vi "Statistics.vi"(11 "input data":dbl[](array[numeric])=[4.507, 5.12, 4.497, 5.011, 3.613, 3.857, 5.086, 3.732, 3.995, 3.022, 4.463, 4.377]) -> ()   [LabVIEW 2018]
doc: "This example shows the results of statistical functions. There is a Histogram of all values and there is the Minimum, Maximum and Mean for each packet of data.\n\nThis example uses the following Express VIs: Simulate Signal, Create Histogram, and Statistics."
uses:
  <vilib>/Utility/file.llb/Read Delimited Spreadsheet (DBL).vi
  Instance           2 18Saved   Statistics .vi
  Instance           3 18Saved   Statistics .vi
panel:
  out "subarray 2":dbl[](array[numeric])
  out "subarray":dbl[][](array[numeric])
  in  "length":i32
  in  "index 2":i32
  in  "index":i32
  out "Chart":dynamicdata(graph)
  out "Mean":dbl
  out "Minimum":dbl
  out "Maximum":dbl
  out "Signal":dynamicdata(graph)
  out "Histogram":dynamicdata(graph)
  in  "Stop":bool
  # "Overview: Shows the results of the Statistics Express VI.\nRequirements: LabVIEW Full Development System\nInstructions:\n1. Run the VI.\n2. View the simulated signal (Gaussian noise).\n3. There is a histogram of all values. The chart displays the minimum, maximum and mean for each packet of data.\n4. Click Stop to stop the VI."
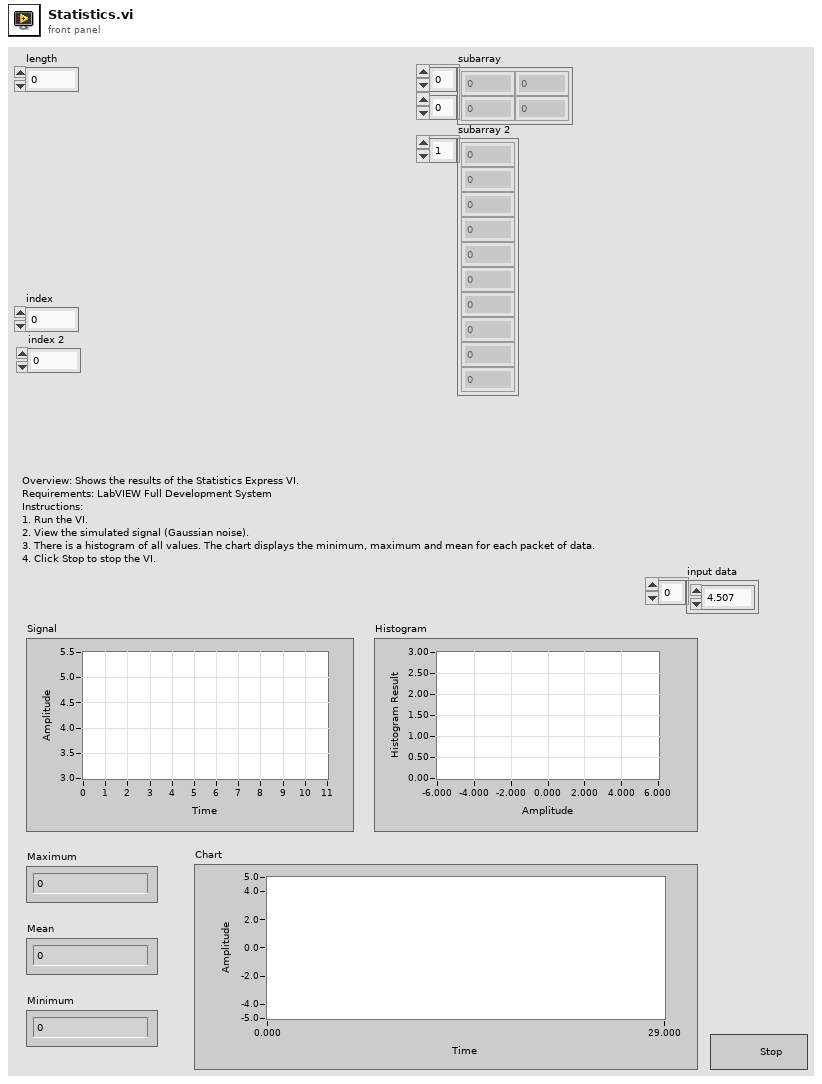
[diagram p1: front panel]
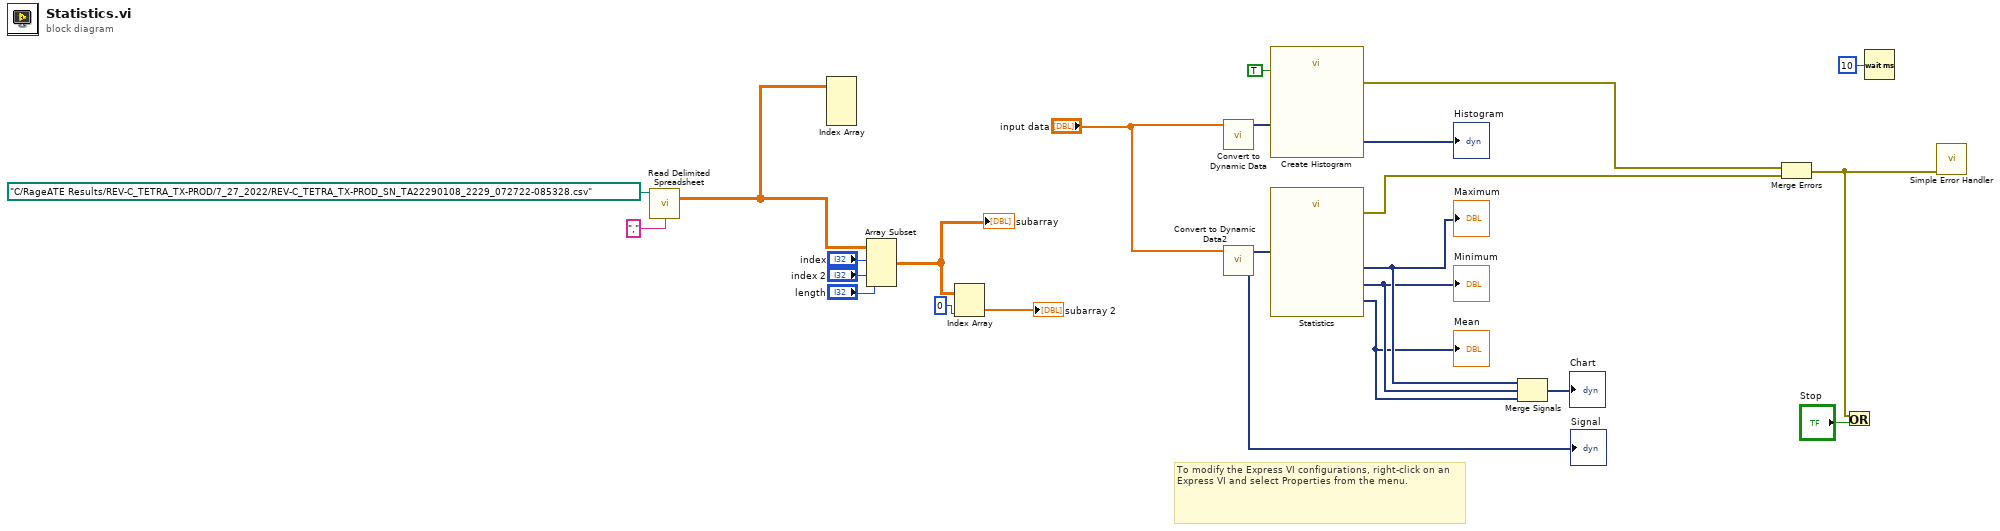
[diagram p0: block diagram]
diagram:
  # "To modify the Express VI configurations, right-click on an Express VI and select Properties from the menu."
  n1 = call-poly <vilib>:"Read Delimited Spreadsheet.vi"("file path (dialog if empty)"=path "C:/RageATE Results/REV-C_TETRA_TX-PROD/7_27_2022/REV-C_TETRA_TX-PROD_SN_TA22290108_2229_072722-085328.csv", "delimiter (\\t)"="," ("delimiter (\\t)")) -> ("all rows"=w3:dbl[][])  [unwired: 8 in, 5 out]
  n2 = Index Array(array=w3) -> ()  [unwired: 4 in, 2 out]
  n3 = Array Subset(array=w3, index (row)="index", index (col)="index 2", length (col)="length") -> (w18:dbl[][])  [unwired: 1 in]
  "subarray" <- w18
  n4 = Index Array(array=w18, index (col)=0 ("index (row)")) -> (element=→"subarray 2":dbl[])  [unwired: 1 in]
  n5 = call "Convert to Dynamic Data"("Array"="input data") -> ("Dynamic Data Type"=w5:dynamicdata)  [unwired: 3 in]
  n6 = call "Convert to Dynamic Data2"("Array"="input data") -> ("Dynamic Data Type"=w4:dynamicdata)  [unwired: 3 in]
  "Signal" <- w4
  n7 = call "Create Histogram"("Reset"=TRUE, "Signal"=w5) -> ("error out"=w8:errorcluster, "Histogram"=→"Histogram":dynamicdata)  [unwired: 8 in]
  n8 = call "Statistics"("Signals"=w4) -> ("Arithmetic Mean"=w10:dynamicdata, "Minimum"=w11:dynamicdata, "Maximum"=w12:dynamicdata, "error out"=w7:errorcluster)  [unwired: 23 in]
  "Maximum" <- w12
  "Minimum" <- w11
  "Mean" <- w10
  n9 = Merge Signals(w12, w11, w10) -> (→"Chart":dynamicdata)
  n10 = Merge Errors(w8, w7) -> (w16:errorcluster)
  n11 = Or(x=w16, y="Stop") -> ()  [unwired: 1 out]
  n12 = Wait (ms)(milliseconds to wait=u32 10) -> ()  [unwired: 1 out]
  n13 = call <vilib>:"Simple Error Handler.vi"("error in (no error)"=w16) -> ()  [unwired: 4 in, 5 out]
